vi "pixelfly_update_status.vi"(8 "error in (no error)":errorcluster, 9 "PixelFly Status Input":T1 {"CCD temp" scale=0.0..100.0; "Board Parameters"."Vertical bin" items=["1", "2"]; "Board Parameters"."Horizontal bin" items=["1", "2"]}, 10 "Acquitsition Settings":T2) -> (0 "error out":errorcluster, 1 "PixelFly Status Output":T1 {"CCD temp" scale=0.0..100.0; "Board Parameters"."Vertical bin" items=["1", "2"]; "Board Parameters"."Horizontal bin" items=["1", "2"]})   [LabVIEW 2016]
uses:
  Controls/PixelFly/PixelFly Status Indicator.ctl
  Controls/PixelFly/Acquisition Settings.ctl
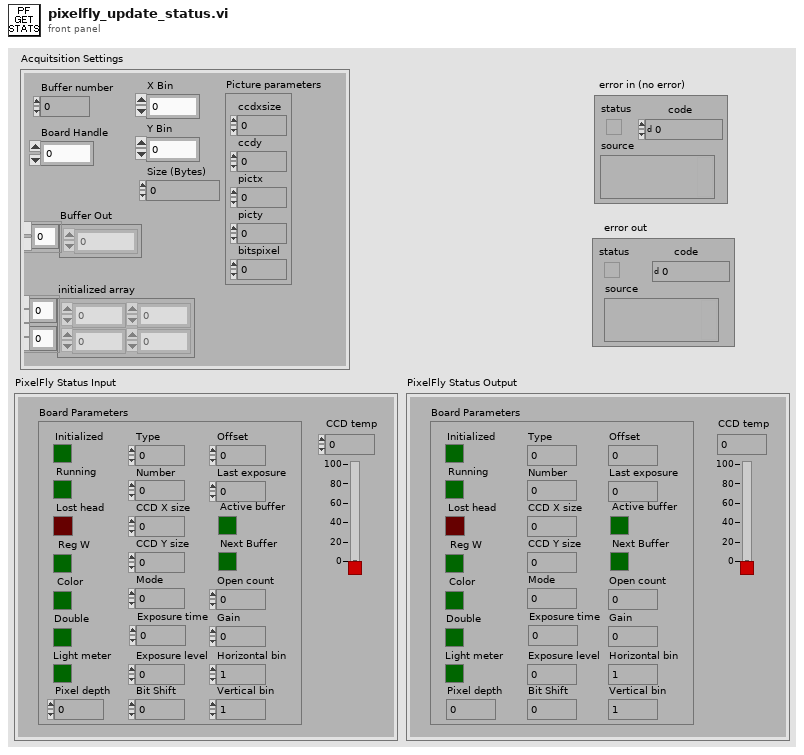
[diagram p1: front panel]
types:
  T1 = typedef "PixelFly Status Indicator.ctl" = cluster{"Board Parameters":cluster{"Type":u32, "Number":u32, "Initialized":bool, "Running":bool, "Lost head":bool, "CCD X size":u32, "CCD Y size":u32, "Mode":u32, "Exposure time":u32, "Exposure level":u32, "Horizontal bin":u32, "Vertical bin":u32, "Reg W":bool, "Gain":u32, "Pixel depth":i32, "Bit Shift":u32, "Offset":u32, "Last exposure":u32, "Double ":bool, "Light meter":bool, "Color":bool, "Open count":u32, "Active buffer":bool, "Next Buffer":bool}, "CCD temp":i32}
  T2 = typedef "Acquisition Settings.ctl" = cluster{"Buffer number":i32, "Size (Bytes)":i32, "initialized array":u16[][], "X Bin":i32, "Y Bin":i32, "Board Handle":u32, "Picture parameters":cluster{"ccdxsize":i32, "ccdy":i32, "pictx":i32, "picty":i32, "bitspixel":i32}, "Buffer Out":u16[]}
  T3 = cluster{"Type":u32, "Number":u32, "Initialized":bool, "Running":bool, "Lost head":bool, "CCD X size":u32, "CCD Y size":u32, "Mode":u32, "Exposure time":u32, "Exposure level":u32, "Horizontal bin":u32, "Vertical bin":u32, "Reg W":bool, "Gain":u32, "Pixel depth":i32, "Bit Shift":u32, "Offset":u32, "Last exposure":u32, "Double ":bool, "Light meter":bool, "Color":bool, "Open count":u32, "Active buffer":bool, "Next Buffer":bool}
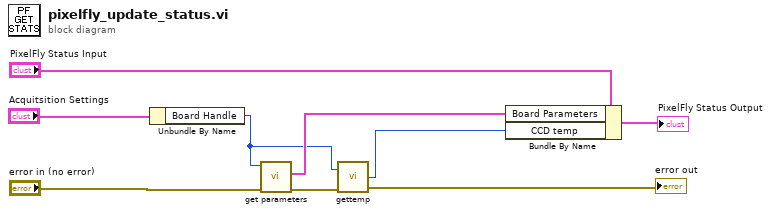
[diagram p0: block diagram]
diagram:
  n1 = Unbundle By Name("Acquitsition Settings") -> ("Board Handle"=w1:u32)
  n2 = call "get parameters.vi"("error in (no error)"="error in (no error)", "Handle in"=w1) -> ("error out"=w9:errorcluster, "Board Parameters"=w4:T3)  [unwired: 2 in, 2 out]
  n3 = call "gettemp.vi"("Handle in"=w1, "error in (no error)"=w9) -> ("ccdtemp"=w5:i32, "error out"=→"error out":errorcluster)  [unwired: 1 out]
  n4 = Bundle By Name(cluster="PixelFly Status Input", "Board Parameters"=w4, "CCD temp"=w5) -> (→"PixelFly Status Output":T1)
